vi "resultCompare.vi"(2 "P2":dbl, 4 "P1":dbl) -> (1 "result":string)   [LabVIEW 2014]
doc: "Compares the result to mark the winner, or if it is a tie game."
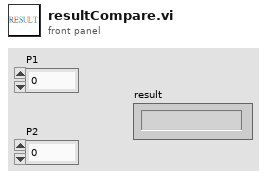
[diagram p1: front panel]
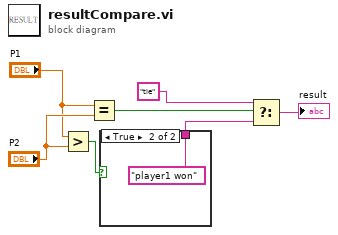
[diagram p0: block diagram]
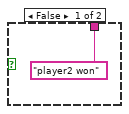
[diagram p2: hidden frame]
diagram:
  n1 = Greater?(x="P1", y="P2") -> (0:w3:bool)
  n2 = Equal?(x="P1", y="P2") -> (x = y?=w7:bool)
  n3 = case shown="True" w3 {
    tunnel: ["player2 won" "player1 won"] -> w2
    frame False {
    }
    frame True {
    }
  }
  n4 = Select(t="tie", s=w7, f=w2) -> (s? t:f=→"result":string)
